vi "dataProcess_coherenceLength.vi"(0 "reference":refnum<class "OSA200.lvclass">, 1 "samplesPerRefPeriod":sgl, 2 "interferogram":sgl[](array[numeric]), 3 "X min interferogram (cm)":sgl, 4 "X max interferogram (cm)":sgl, 5 "error in (no error)":errorcluster, 6 "X range":T1(ring), 8 "X min (cm)":sgl format="%.2f", 10 "X max (cm)":sgl format="%.2f") -> (14 "duplicate reference":refnum<class "OSA200.lvclass">, 15 "coherence length error(cm)":dbl, 16 "coherence length (cm)":dbl, 19 "error out":errorcluster)   [LabVIEW 2010, in "OSA200.lvclass"]
doc: "Estimates the coherence length of the input light source by analyzing the interferogram.\n\nThis vi calls FTS_CoherenceLength_Array, (FTSLib.dll), with the interferogram input parameter pointing to the interferogram control data of this vi or, if empty, to the labview interferogram buffer. \n\nSee buffer_get.vi or trace_toLVBuffer.vi for OSA200 labview buffer handling."
uses:
  OSA200.lvclass
  OSA.lvclass
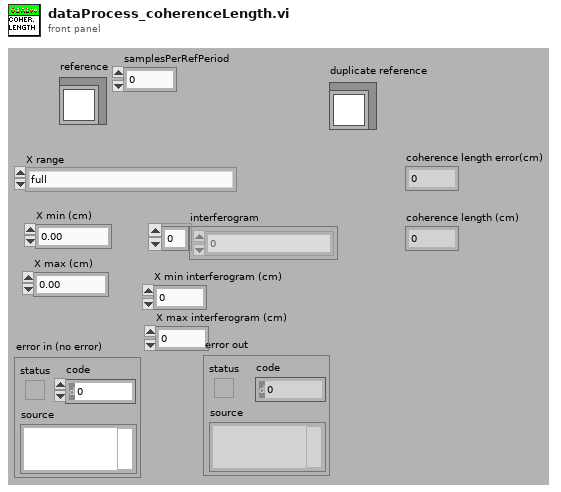
[diagram p1: front panel]
types:
  T1 = enum16{"full", "zero symmetric (-X min .... +X min)", "zero asymmetric (X min .... X max)"}
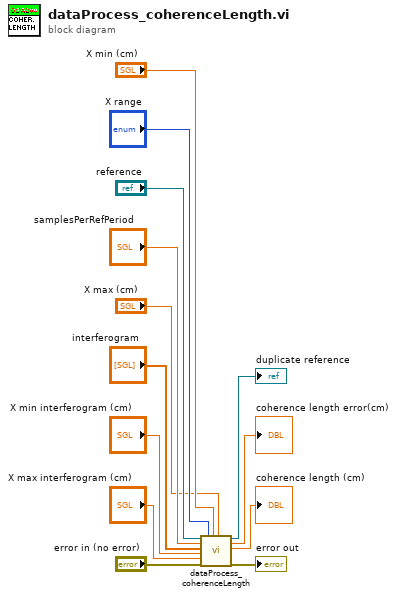
[diagram p0: block diagram]
diagram:
  n1 = call-parent "dataProcess_coherenceLength.vi"("reference"="reference", "samplesPerRefPeriod"="samplesPerRefPeriod", "interferogram"="interferogram", "X min interferogram (cm)"="X min interferogram (cm)", "X max interferogram (cm)"="X max interferogram (cm)", "error in (no error)"="error in (no error)", "X range"="X range", "X min (cm)"="X min (cm)", "X max (cm)"="X max (cm)") -> ("duplicate reference"=→"duplicate reference":refnum<class "OSA200.lvclass">, "coherence length error(cm)"=→"coherence length error(cm)":dbl, "coherence length (cm)"=→"coherence length (cm)":dbl, "error out"=→"error out":errorcluster)  [unwired: 7 in]
